vi "Mod_OFDM_Set_Ofdm_Parameters.vi"(0 "Configuration in":variant, 7 "OFDM Parameters":T1={"# of Sub Carrier"=15, "Length Of Cylic Prefix"=3}, 11 "error in":errorcluster) -> (4 "Configuration out":variant, 15 "error out":errorcluster)   [LabVIEW 2010]
uses:
  Mod_OFDM_Get_Sub_Carrier_Selection.vi
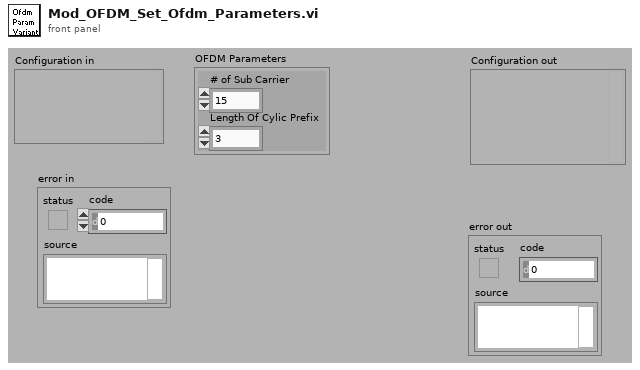
[diagram p1: front panel]
types:
  T1 = cluster{"# of Sub Carrier":i32, "Length Of Cylic Prefix":i32}
  T2 = cluster{"Sub Carrier Selection":cluster{"Sub Carrier":bool, "Data Source":u16, "Modulator":u16}[], "OFDM Parameters":cluster{"# of Sub Carrier":i32, "Length Of Cylic Prefix":i32}}
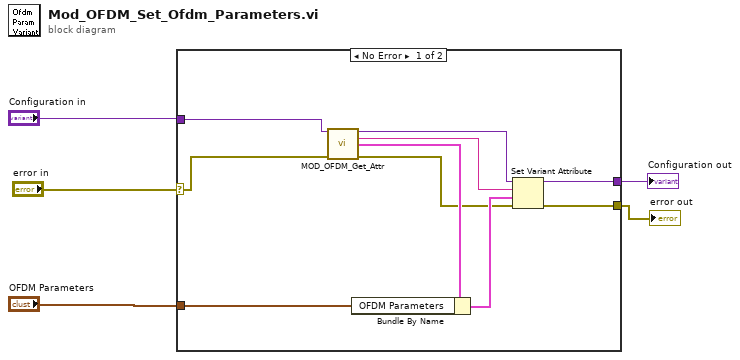
[diagram p0: block diagram]
diagram:
  n1 = case shown="No Error" "error in" {
    selector: "error in" -> [w9 w16]
    tunnel: [w15 w16] -> w5
    tunnel: [w14 _] -> w4
    tunnel: "OFDM Parameters" -> [w11 _]
    tunnel: "Configuration in" -> [w10 _]
    frame No Error {
      n2 = call-poly "MOD_OFDM_Get_Attr.vi"("Configure Variant"=w10, "error in"=w9) -> ("Configure Variant"=w13:variant, 6:"Sub Carrier Selection"=w6:string, 8:"Sub Carrier Selection"=w8:T2, "error out"=w7:errorcluster)  [unwired: 10 in]
      n3 = Bundle By Name(cluster=w8, "OFDM Parameters"=w11) -> (w12:T2)
      n4 = Set Variant Attribute(Variant=w13, name=w6, value=w12, error in=w7) -> (Variant out=w14:variant, error out=w15:errorcluster)  [unwired: 1 out]
    }
    frame Error {
    }
  }
  "error out" <- w5
  "Configuration out" <- w4
